vi "AlliGator Check Background Dataset Compatibility.vi"(8 "Background Image Loading Options":T4 {"Hot Pixel Removal"."Percentile" min=0 max=100; "Image Binning Options"."Y Bin" min=1; "Image Binning Options"."X Bin" min=1; "Image Smoothing Options"."Bin" min=1}, 9 "Background FLI Data File Information":T1, 10 "Dataset Image Loading Options":T4 {"Hot Pixel Removal"."Percentile" min=0 max=100; "Image Binning Options"."Y Bin" min=1; "Image Binning Options"."X Bin" min=1; "Image Smoothing Options"."Bin" min=1}, 11 "Dataset FLI Data File Information":T1) -> (0 "Error Out":errorcluster, 3 "Compatible Background Dataset?":bool)   [LabVIEW 2021, in "AlliGator Files.lvlib"]
doc: "Compares settings of FLI dataset and background dataset to check for tueir compatibility."
uses:
  AlliGator Files.lvlib
  AlliGator Image Loading Options.ctl
  AlliGator Image Smoothing Options.ctl
  Arrays/Kernel Type.ctl
  Arrays/Smoothing Algorithm.ctl
  AlliGator Gates to Skip.ctl
  AlliGator Image Binning Options.ctl
  AlliGator Gates to Keep.ctl
  SwissSPAD/SwissSPAD Live_Image Display Options.ctl
  AlliGator Image Pre-processing Step.ctl
  AlliGator FLI Data File Information.ctl
  Phasor/Phasor Fluorescence Lifetime Parameters v3.ctl
  AlliGator FLI Dataset Type.ctl
  f7ee2ffc-540b-4f59-982f-e209fcab6e3f.vi
  3bae9903-ba0c-4aea-b0f8-08fc38513d17.vi
  b01e33b0-9348-48e9-a498-30259952dc97.vi
  53257ff1-e046-4ef1-8fbc-2a820b3c694c.vi
  f7ee2ffc-540b-4f59-982f-e209fcab6e3f.vi/8a80743f-1319-44c8-96b0-3ef8fc688731.vi
  f7ee2ffc-540b-4f59-982f-e209fcab6e3f.vi/931f4f8f-d8c6-4056-833f-5c8fe97b24b9.vi
  3bae9903-ba0c-4aea-b0f8-08fc38513d17.vi/8a80743f-1319-44c8-96b0-3ef8fc688731.vi
  3bae9903-ba0c-4aea-b0f8-08fc38513d17.vi/931f4f8f-d8c6-4056-833f-5c8fe97b24b9.vi
  b01e33b0-9348-48e9-a498-30259952dc97.vi/8a80743f-1319-44c8-96b0-3ef8fc688731.vi
  b01e33b0-9348-48e9-a498-30259952dc97.vi/931f4f8f-d8c6-4056-833f-5c8fe97b24b9.vi
  53257ff1-e046-4ef1-8fbc-2a820b3c694c.vi/8a80743f-1319-44c8-96b0-3ef8fc688731.vi
  53257ff1-e046-4ef1-8fbc-2a820b3c694c.vi/931f4f8f-d8c6-4056-833f-5c8fe97b24b9.vi
  <vilib>/Utility/error.llb/Error Cluster From Error Code.vi
  <vilib>/ErrorRing/Error Ring.xnode
  Strings/Strings.lvlib
  Notebook/Notebook.lvlib
  Rich Text Box/Rich Text Box.lvlib
  Error/Error.lvlib
  Arrays/Arrays.lvlib
  AlliGator Settings.lvlib
  AlliGator Decay Analysis.lvlib
  AlliGator Source Image.lvlib
  AlliGator HDF5.lvlib
  SwissSPAD/SwissSPAD Live.lvlib
  Phasor/Phasor.lvlib
panel:
  # "see the AlliGator License on the block diagram (Ctrl+E or Window:Show Block Diagram)"
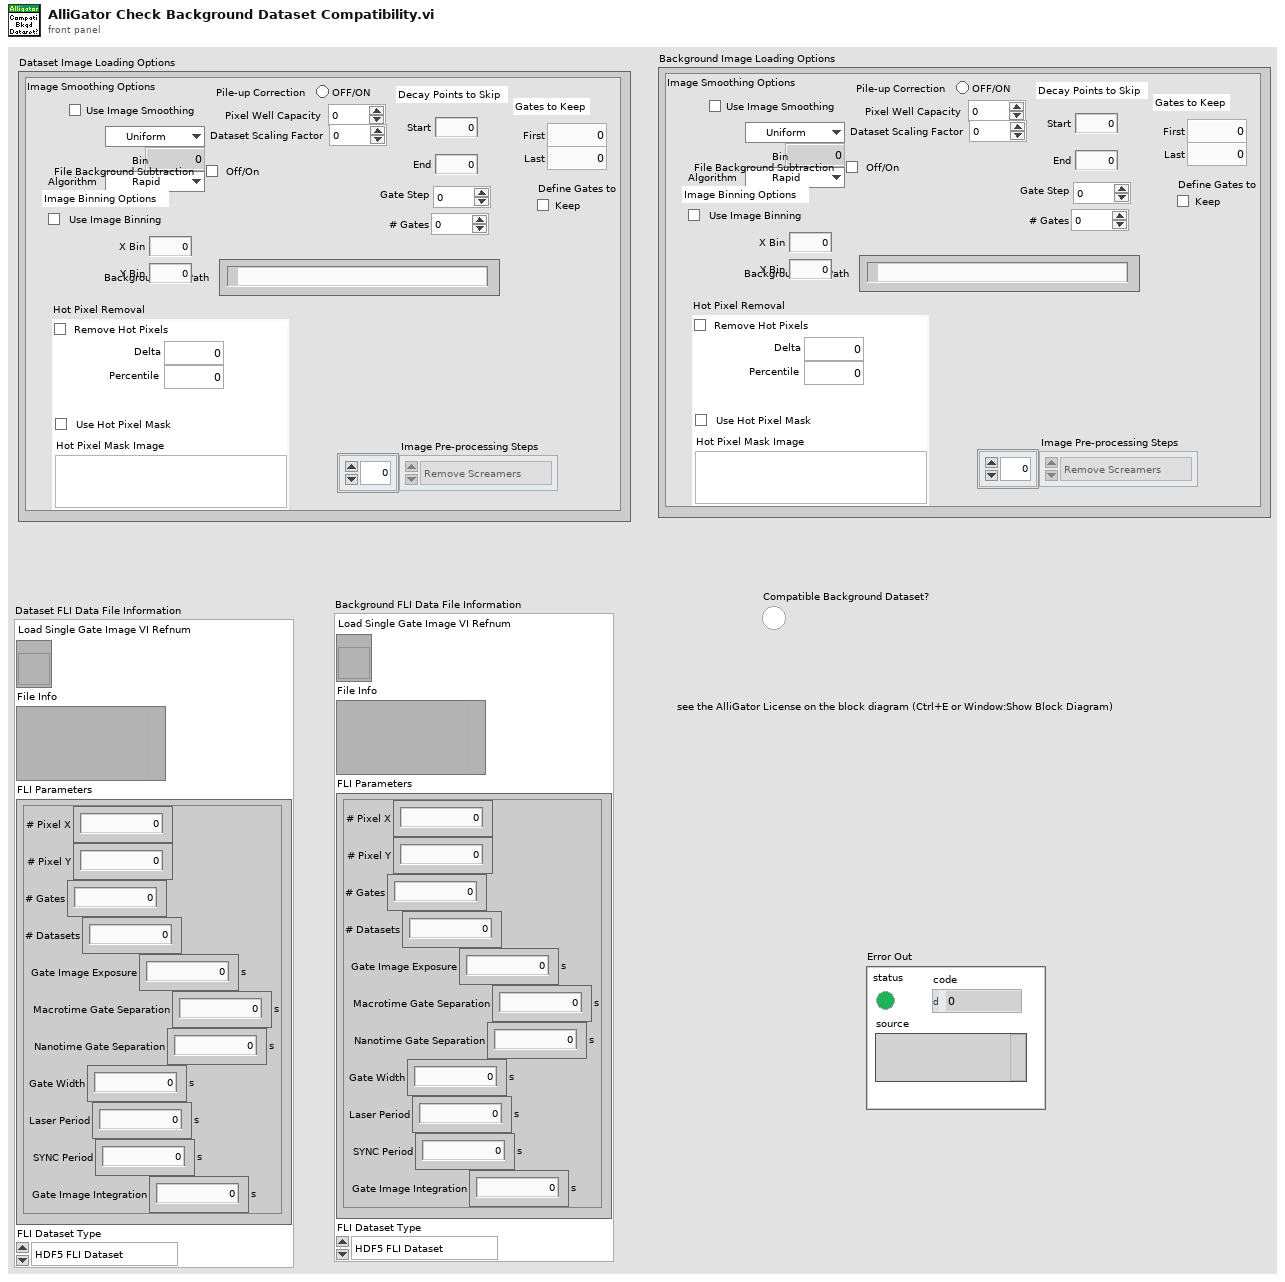
[diagram p1: front panel]
types:
  T1 = typedef "AlliGator HDF5.lvlib/AlliGator FLI Data File Information.ctl" = cluster{"Load Single Gate Image VI Refnum":refnum<vi>, "File Info":variant, "FLI Parameters":T2, "FLI Dataset Type":T3}
  T2 = typedef "Phasor.lvlib/Phasor Fluorescence Lifetime Parameters v3.ctl" = cluster{"# Pixel X":i32, "# Pixel Y":i32, "# Gates":i32, "# Datasets":i32, "Gate Image Exposure":dbl[unit], "Macrotime Gate Separation":dbl[unit], "Nanotime Gate Separation":dbl[unit], "Gate Width":dbl[unit], "Laser Period":dbl[unit], "SYNC Period":dbl[unit], "Gate Image Integration":dbl[unit]}
  T3 = typedef "AlliGator Files.lvlib/AlliGator FLI Dataset Type.ctl" = enum16{"HDF5 FLI Dataset", "Gate Image Folder", ".sdt FLI Dataset (Becker & Hickl)", ".ptu FLI Dataset (PicoQuant)", "SS1 FLI Dataset", "SS2 FLI Dataset", "I/m/phi Dataset", ".bin FLI Dataset (PicoQuant Binned)", ".bin FLI Dataset (Piccolo Binned)"}
  T4 = typedef "AlliGator Source Image.lvlib/AlliGator Image Loading Options.ctl" = cluster{"Pixel Well Capacity":u32, "Pile-up Correction":bool, "Gate Step":i32, "Image Smoothing Options":T5, "Gates to Skip":T8, "File Background Subtraction":bool, "Background File Path":path, "Image Binning Options":T9, "# Gates":u32, "Gates to Keep":T10, "Define Gates to":bool, "Hot Pixel Removal":T11, "Dataset Scaling Factor":dbl, "Image Pre-processing Steps":T12[]}
  T5 = typedef "AlliGator Settings.lvlib/AlliGator Image Smoothing Options.ctl" = cluster{"Use Image Smoothing":bool, "Kernel Type":T6, "Bin":i32, "Algorithm":T7}
  T6 = typedef "Arrays.lvlib/Kernel Type.ctl" = enum16{"Uniform", "Bilinear", "Gaussian"}
  T7 = typedef "Arrays.lvlib/Smoothing Algorithm.ctl" = enum16{"Rapid", "Thorough"}
  T8 = typedef "AlliGator Decay Analysis.lvlib/AlliGator Gates to Skip.ctl" = cluster{"Start":u32, "End":u32}
  T9 = typedef "AlliGator Source Image.lvlib/AlliGator Image Binning Options.ctl" = cluster{"Use Image Binning":bool, "X Bin":i32, "Y Bin":i32}
  T10 = typedef "AlliGator Settings.lvlib/AlliGator Gates to Keep.ctl" = cluster{"First":u32, "Last":u32}
  T11 = typedef "SwissSPAD Live.lvlib/SwissSPAD Live_Image Display Options.ctl" = cluster{"Remove Screamers":bool, "Delta":sgl, "Equalize Histogram":bool, "Percentile":sgl, "Hot Pixel Mask Image":path, "Use Hot Pixel Mask":bool}
  T12 = typedef "AlliGator Files.lvlib/AlliGator Image Pre-processing Step.ctl" = enum16{"Remove Screamers", "Pile-up Correction", "Binning", "Smoothing", "Rescaling", "Dead Left Column Correction"}
  T13 = cluster{"Pixel Well Capacity":bool, "Pile-up Correction":bool, "Gate Step":bool, "Image Smoothing Options":cluster{"Use Image Smoothing":bool, "Kernel Type":bool, "Bin":bool, "Algorithm":bool}, "Gates to Skip":cluster{"Start":bool, "End":bool}, "File Background Subtraction":bool, "Background File Path":bool, "Image Binning Options":cluster{"Use Image Binning":bool, "X Bin":bool, "Y Bin":bool}, "# Gates":bool, "Gates to Keep":cluster{"First":bool, "Last":bool}, "Define Gates to":bool, "Hot Pixel Removal":cluster{"Remove Screamers":bool, "Delta":bool, "Equalize Histogram":bool, "Percentile":bool, "Hot Pixel Mask Image":bool, "Use Hot Pixel Mask":bool}, "Dataset Scaling Factor":bool, "Image Pre-processing Steps":bool[]}
  T14 = cluster{"Use Image Binning":bool, "X Bin":bool, "Y Bin":bool}
  T15 = typedef "Rich Text Box.lvlib/Text Formatting.ctl" = cluster{"Font":string, "Text Color":T16, "Text Background Color":T16, "Text Style":enum16{"Regular", "Bold", "Italic", "Underline", "Strikeout"}, "Font Size (Points)":dbl, "Text Alignment":i32}
  T16 = typedef "Rich Text Box.lvlib/Text Colors.ctl" = enum16{"Unchanged", "Black", "Blue", "Brown", "Gray", "Green", "Orange", "Pink", "Red", "White"}
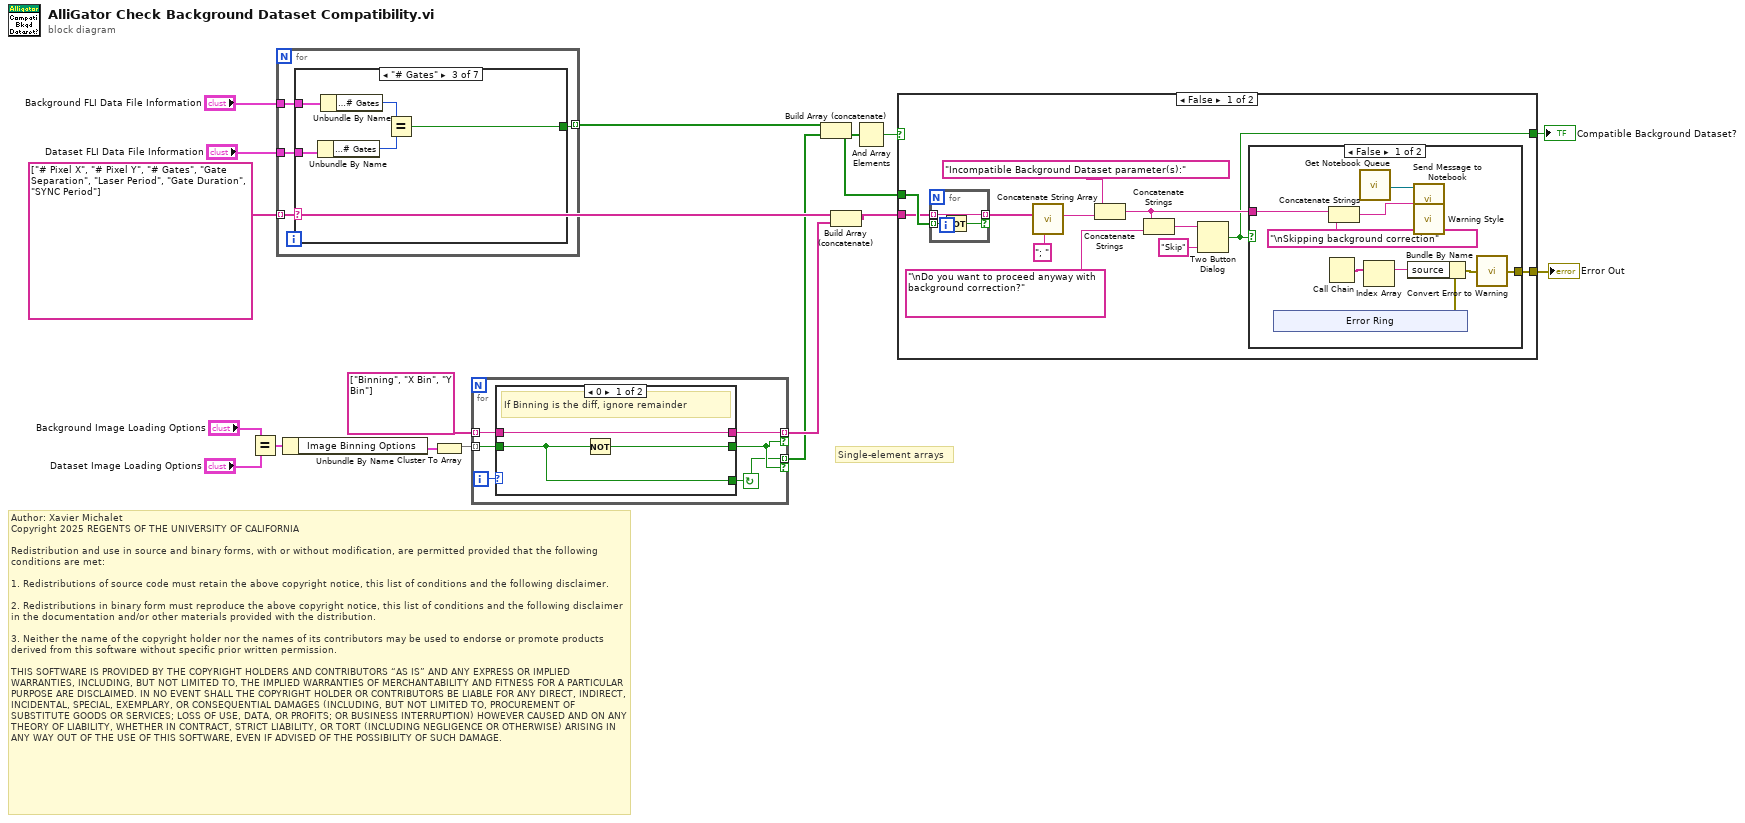
[diagram p0: block diagram]
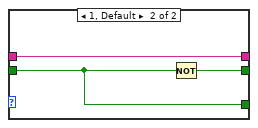
[diagram p2: hidden frame]
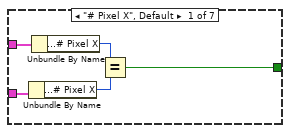
[diagram p5: hidden frame]
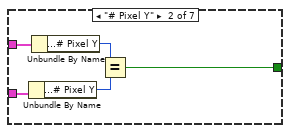
[diagram p6: hidden frame]
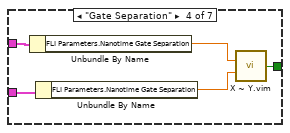
[diagram p7: hidden frame]
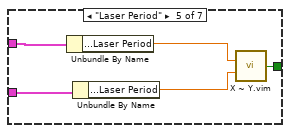
[diagram p8: hidden frame]
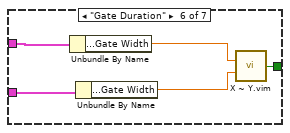
[diagram p9: hidden frame]
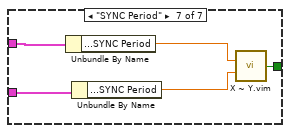
[diagram p10: hidden frame]
diagram:
  w6 = string[] ["# Pixel X", "# Pixel Y", "# Gates", "Gate Separation", "Laser Period", "Gate Duration", "SYNC Period"]
  # "Single-element arrays"
  # "Author: Xavier Michalet\nCopyright 2025 REGENTS OF THE UNIVERSITY OF CALIFORNIA\n\nRedistribution and use in source and binary forms, with or without modification, are permitted provided that the following conditions are met:\n\n1. Redistributions of source code must retain the above copyright notice, this list of conditions and the following disclaimer.\n\n2. Redistributions in binary form must reproduce the above copyright notice, this list of conditions and the following disclaimer in the documentation and/or other materials provided with the distribution.\n\n3. Neither the name of the copyright holder nor the names of its contributors may be used to endorse or promote products derived from this software without specific prior written permission.\n\nTHIS SOFTWARE IS PROVIDED BY THE COPYRIGHT HOLDERS AND CONTRIBUTORS “AS IS” AND ANY EXPRESS OR IMPLIED WARRANTIES, INCLUDING, BUT NOT LIMITED TO, THE IMPLIED WARRANTIES OF MERCHANTABILITY AND FITNESS FOR A PARTICULAR PURPOSE ARE DISCLAIMED. IN NO EVENT SHALL THE COPYRIGHT HOLDER OR CONTRIBUTORS BE LIABLE FOR ANY DIRECT, INDIRECT, INCIDENTAL, SPECIAL, EXEMPLARY, OR CONSEQUENTIAL DAMAGES (INCLUDING, BUT NOT LIMITED TO, PROCUREMENT OF SUBSTITUTE GOODS OR SERVICES; LOSS OF USE, DATA, OR PROFITS; OR BUSINESS INTERRUPTION) HOWEVER CAUSED AND ON ANY THEORY OF LIABILITY, WHETHER IN CONTRACT, STRICT LIABILITY, OR TORT (INCLUDING NEGLIGENCE OR OTHERWISE) ARISING IN ANY WAY OUT OF THE USE OF THIS SOFTWARE, EVEN IF ADVISED OF THE POSSIBILITY OF SUCH DAMAGE."
  n1 = Equal?(x="Background Image Loading Options", y="Dataset Image Loading Options") -> (x = y?=w15:T13)
  n2 = for {
    tunnel: w6 -> [w21] mode=indexing
    tunnel: "Dataset FLI Data File Information" -> [w19]
    tunnel: "Background FLI Data File Information" -> [w20]
    tunnel: [w18] -> w3 mode=indexing
    n3 = case shown="\"# Gates\"" w21 {
      tunnel: w20 -> [w26 w31 w36 w41 w46 w51 w56]
      tunnel: w19 -> [w25 w30 w35 w40 w45 w50 w55]
      tunnel: [w22 w27 w32 w39 w44 w49 w54] -> w18
      frame "# Pixel X", Default {
        n4 = Unbundle By Name(w25) -> ("FLI Parameters.# Pixel X"=w23:i32)
        n5 = Unbundle By Name(w26) -> ("FLI Parameters.# Pixel X"=w24:i32)
        n6 = Equal?(x=w24, y=w23) -> (x = y?=w22:bool)
      }
      frame "# Pixel Y" {
        n7 = Unbundle By Name(w30) -> ("FLI Parameters.# Pixel Y"=w28:i32)
        n8 = Unbundle By Name(w31) -> ("FLI Parameters.# Pixel Y"=w29:i32)
        n9 = Equal?(x=w29, y=w28) -> (x = y?=w27:bool)
      }
      frame "# Gates" {
        n10 = Unbundle By Name(w35) -> ("FLI Parameters.# Gates"=w33:i32)
        n11 = Unbundle By Name(w36) -> ("FLI Parameters.# Gates"=w34:i32)
        n12 = Equal?(x=w34, y=w33) -> (x = y?=w32:bool)
      }
      frame "Gate Separation" {
        n13 = Unbundle By Name(w41) -> ("FLI Parameters.Nanotime Gate Separation"=w38:dbl[unit])
        n14 = Unbundle By Name(w40) -> ("FLI Parameters.Nanotime Gate Separation"=w37:dbl[unit])
        n15 = call "X ~ Y.vim"("X"=w38, "Y"=w37) -> ("X ~= Y?"=w39:bool)  [unwired: 13 in]
      }
      frame "Laser Period" {
        n16 = Unbundle By Name(w46) -> ("FLI Parameters.Laser Period"=w43:dbl[unit])
        n17 = Unbundle By Name(w45) -> ("FLI Parameters.Laser Period"=w42:dbl[unit])
        n18 = call "X ~ Y.vim"("X"=w43, "Y"=w42) -> ("X ~= Y?"=w44:bool)  [unwired: 13 in]
      }
      frame "Gate Duration" {
        n19 = Unbundle By Name(w51) -> ("FLI Parameters.Gate Width"=w48:dbl[unit])
        n20 = Unbundle By Name(w50) -> ("FLI Parameters.Gate Width"=w47:dbl[unit])
        n21 = call "X ~ Y.vim"("X"=w48, "Y"=w47) -> ("X ~= Y?"=w49:bool)  [unwired: 13 in]
      }
      frame "SYNC Period" {
        n22 = Unbundle By Name(w56) -> ("FLI Parameters.SYNC Period"=w53:dbl[unit])
        n23 = Unbundle By Name(w55) -> ("FLI Parameters.SYNC Period"=w52:dbl[unit])
        n24 = call "X ~ Y.vim"("X"=w53, "Y"=w52) -> ("X ~= Y?"=w54:bool)  [unwired: 13 in]
      }
    }
  }
  n25 = Unbundle By Name(w15) -> ("Image Binning Options"=w14:T14)
  n26 = Cluster To Array(cluster=w14) -> (array=w10:bool[])
  n27 = for {
    tunnel: w10 -> [w60] mode=indexing
    tunnel: [w61] -> w7 mode=indexing if=w58
    tunnel: string[] ["Binning", "X Bin", "Y Bin"] -> [w59] mode=indexing
    tunnel: [w57] -> w1 mode=indexing if=w58
    i -> [w62]
    stop <- w57 continue-if-true
    n28 = case shown="0" w62 {
      tunnel: [w63 w68] -> w61
      tunnel: [w65 w67] -> w58
      tunnel: w60 -> [w64 w66]
      tunnel: [w64 w66] -> w57
      tunnel: w59 -> [w63 w68]
      frame 0 {
        # "If Binning is the diff, ignore remainder"
        n29 = Not(x=w64) -> (.not. x?=w65:bool)
      }
      frame 1, Default {
        n30 = Not(x=w66) -> (.not. x?=w67:bool)
      }
    }
  }
  n31 = Build Array (concatenate)(w3, w1) -> (w11:bool[])
  n32 = Build Array (concatenate)(w6, w7) -> (w8:string[])
  n33 = And Array Elements(Boolean array=w11) -> (logical AND=w12:bool)
  n34 = case shown="False" w12 {
    selector: w12 -> [_ w98]
    tunnel: [w71 _] -> w13
    tunnel: w11 -> [w80 _]
    tunnel: w8 -> [w79 _]
    tunnel: [w69 w98] -> w2
    frame False {
      n35 = for {
        tunnel: w80 -> [w96] mode=indexing
        tunnel: w79 -> [w97] mode=indexing
        tunnel: [w97] -> w78 mode=indexing if=w95
        n36 = Not(x=w96) -> (.not. x?=w95:bool)
      }
      n37 = call "Concatenate String Array.vi"("Separator (TAB)"="; ", "String Array"=w78) -> ("Formatted String"=w76:string)  [unwired: 9 in]
      n38 = Concatenate Strings("Incompatible Background Dataset parameter(s):" ("Prefix (\"\")"), w76) -> (w70:string)
      n39 = Concatenate Strings(w70, "\nDo you want to proceed anyway with background correction?" ("string")) -> (w73:string)
      n40 = Two Button Dialog(message=w73, 1:"Skip" ("F button name (\"Cancel\")")) -> (T button?=w69:bool)  [unwired: 1 in]
      n41 = case shown="False" w69 {
        tunnel: [w84 _] -> w71
        tunnel: w70 -> [w83 _]
        frame False {
          n42 = xnode "Error Ring"() -> ("error out"=w90:errorcluster)
          n43 = Call Chain() -> (call chain=w88:string[])
          n44 = Concatenate Strings(w83, "\nSkipping background correction" ("Suffix (\"\")")) -> (w81:string)
          n45 = call "Get Notebook Queue.vi"() -> ("Notebook Queue"=w86:refnum<queue>)  [unwired: 9 in]
          n46 = Index Array(array=w88) -> (element=w87:string)  [unwired: 1 in]
          n47 = Bundle By Name(cluster=w90, "source"=w87) -> (w89:errorcluster)
          n48 = call "Warning Style.vi"() -> ("Error Formatting"=w85:T15)
          n49 = call "Send Message to Notebook.vi"("Text Formatting"=w85, "Message"=w81, "Notebook Queue"=w86) -> ()  [unwired: 5 in, 2 out]
          n50 = call "Convert Error to Warning.vi"("Error In"=w89) -> ("no Error Out"=w84:errorcluster)  [unwired: 8 in]
        }
        frame True {
        }
      }
    }
    frame True {
    }
  }
  "Compatible Background Dataset?" <- w2
  "Error Out" <- w13
